vi "Calculate Temperature Setpoints from GenCal Values.vi"() -> ()   [LabVIEW 2010]
panel:
  out "Temp Offset Abort":dbl
  out "Temp Offset Critical":dbl
  out "Temp Offset Warning":dbl
  out "Temp Offset Minimum":dbl
  in  "Cal Abort Threshold (R/4)":u16 format="%x"
  in  "Cal Critical Threshold (R/4)":u16 format="%x"
  in  "Cal Warning Threshold (R/4)":u16 format="%x"
  in  "Cal Minimum Threshold (R/4)":u16 format="%x"
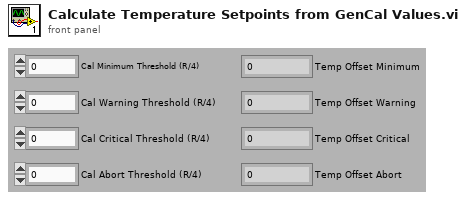
[diagram p1: front panel]
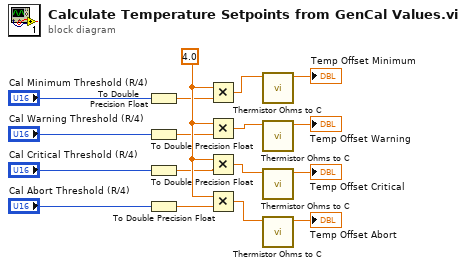
[diagram p0: block diagram]
diagram:
  w17 = 4.0 ("x")
  n1 = To Double Precision Float(number="Cal Minimum Threshold (R/4)") -> (double precision float=w15:dbl)
  n2 = To Double Precision Float(number="Cal Warning Threshold (R/4)") -> (double precision float=w11:dbl)
  n3 = To Double Precision Float(number="Cal Critical Threshold (R/4)") -> (double precision float=w10:dbl)
  n4 = To Double Precision Float(number="Cal Abort Threshold (R/4)") -> (double precision float=w9:dbl)
  n5 = Multiply(x=w17, y=w15) -> (x*y=w4:dbl)
  n6 = Multiply(x=w17, y=w11) -> (x*y=w3:dbl)
  n7 = Multiply(x=w17, y=w10) -> (x*y=w2:dbl)
  n8 = Multiply(x=w17, y=w9) -> (x*y=w1:dbl)
  n9 = call "Thermistor Ohms to C.vi"("Thermistor R"=w4) -> ("Thermistor C"=→"Temp Offset Minimum":dbl)  [unwired: 10 in]
  n10 = call "Thermistor Ohms to C.vi"("Thermistor R"=w3) -> ("Thermistor C"=→"Temp Offset Warning":dbl)  [unwired: 10 in]
  n11 = call "Thermistor Ohms to C.vi"("Thermistor R"=w2) -> ("Thermistor C"=→"Temp Offset Critical":dbl)  [unwired: 10 in]
  n12 = call "Thermistor Ohms to C.vi"("Thermistor R"=w1) -> ("Thermistor C"=→"Temp Offset Abort":dbl)  [unwired: 10 in]
